vi "FrontPanel_RT.vi"() -> ()   [LabVIEW 2015]
uses:
  Classes/MotorControl/TypeDef/MotorMode.ctl
  Classes/CAlex2-Display/CAlex2_Display.lvclass
  Classes/CAlex2/TypeDef/LowerBodyDim.ctl
  Classes/ForceField/TypeDef/FF_Gains.ctl
  Classes/MotorControl/MotorControl.lvclass
  Classes/CAlex2/CAlex2.lvclass
  Classes/SerialChain-Cable/SerialChain-Cable.lvclass
  Classes/ForceField/ForceField.lvclass
  <vilib>/GoldZinc Software/auzn custom VIs/CustomVI.lvlib
panel:
  in  "Motor Mode":T1={"Idle"=FALSE, "Pre"=FALSE, "Pre-Value"=7, "PID"=FALSE} {"Pre-Value" items=["7N"=7, "10N"=10, "15N"=15, "20N"=20]}
  out "ViconConnected":bool
  in  "ResetIMU":bool
  in  "Vicon":bool
  in  "Extra Wt (kg)":cluster{"Thigh":dbl, "Shank":dbl}
  in  "UpdateFF":bool
  in  "XZ":bool
  in  "YZ":bool
  in  "XY":bool
  out "R_Hill":u32(colorbox)
  out "R_Ball":u32(colorbox)
  out "R_Toe":u32(colorbox)
  out "L_Hill":u32(colorbox)
  out "L_Ball":u32(colorbox)
  out "L_Toe":u32(colorbox)
  in  "Status 8":bool
  out "Waveform Chart 8":cluster{"[0]":dbl, "[1]":dbl}(graph)
  in  "Cuff Location":T2={"HipWd"=0.4, "HipHt"=0.1, "ThighDist"=0.0, "ThighToKnee"=0.05, "HipFwd"=0.0, "ShankToKnee"=0.15}
  in  "Force Field":bool
  in  "ArmWeight":bool
  in  "CuffWeight":bool
  out "Normal Force Tunnel Shape":cluster{dbl[], dbl[]}[](graph)
  in  "File Name":string
  out "Record Time":dbl format="%.2f"
  in  "Leg Property":T3={"Thigh"=0.42, "Shank"=0.42, "ShankWt"=0.0, "ThighWt"=0.0, "Hip"=0.32}
  in  "Gains":T4
  in  "Reset":bool
  in  "Stop RT":bool
  in  "Status 7":bool
  in  "Status 6":bool
  in  "Status 5":bool
  in  "Status 4":bool
  in  "Status 3":bool
  in  "Status 2":bool
  in  "Status 1":bool
  out "Waveform Chart 7":cluster{"[0]":dbl, "[1]":dbl}(graph)
  out "Waveform Chart 6":cluster{"[0]":dbl, "[1]":dbl}(graph)
  out "Waveform Chart 5":cluster{"[0]":dbl, "[1]":dbl}(graph)
  out "Waveform Chart 4":cluster{"[0]":dbl, "[1]":dbl}(graph)
  out "Waveform Chart 3":cluster{"[0]":dbl, "[1]":dbl}(graph)
  out "Waveform Chart 2":cluster{"[0]":dbl, "[1]":dbl}(graph)
  out "Waveform Chart":cluster{"[0]":dbl, "[1]":dbl}(graph)
  in  "ZeroPosition":bool
  in  "Path Type":u8(ring) items=["Straight Line", "Circle", "Vertical Wall", "Horizontal Surface", "Endoscope"]
  in  "Record Data?":bool
  out "Planned Tensions":dbl[](array[numeric]) format="%.2f"
  out "Motor Command":dbl[](array[numeric]) format="%.5f"
  out "Ankle Center":dbl[](array[numeric]) format="%.4f"
  out "Force Field":dbl[](array[numeric]) format="%.2f"
  out "Joint Angles":dbl[](array[numeric]) format="%.1f"
  in  "TareIMU":bool
  in  "Leg Position":refnum<k7>(container)
  # "C-ALEX Control Interface V2 \nDeveloped by Xin Jin, ROAR Laboratory, Columbia University"
  # "Leg Pose"
  # "Status Monitor"
  # "Subject Information"
  # "Data Record"
  # "Control Panel"
  # "Foot Switch"
  # "Path Type"
  # "Motor Mode"
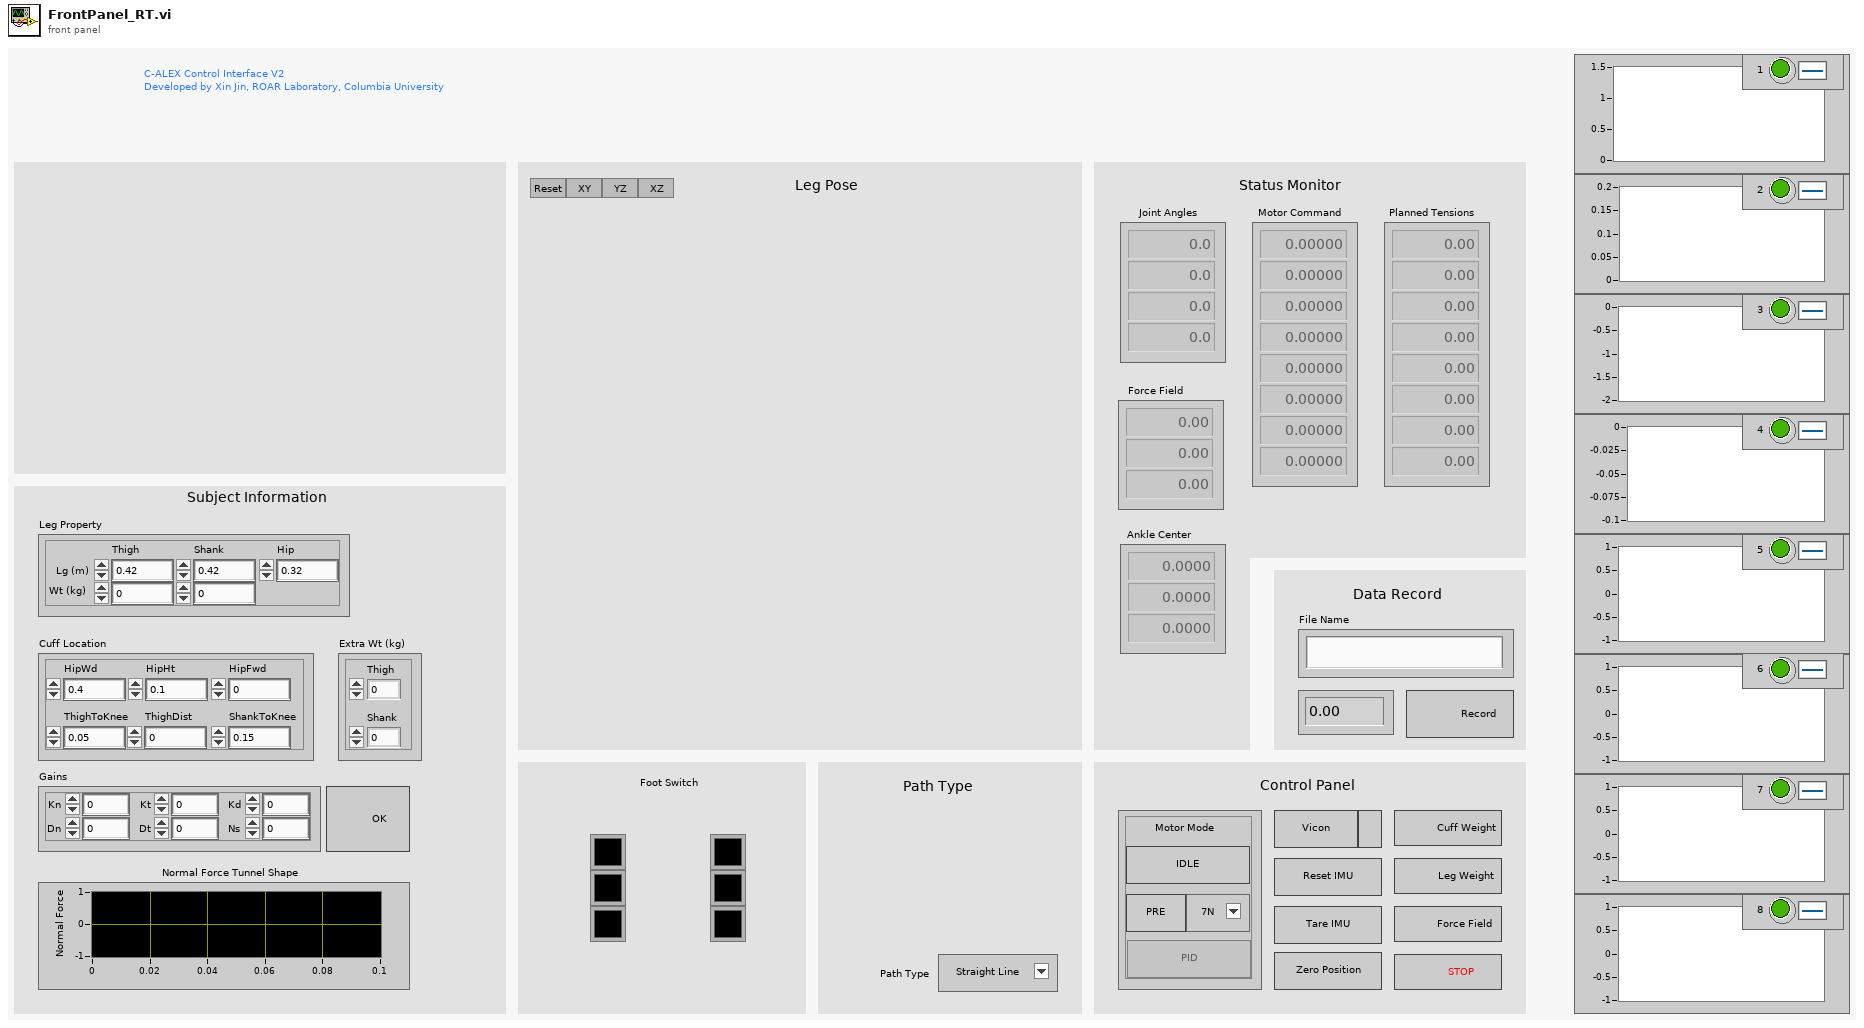
[diagram p1: front panel]
types:
  T1 = cluster{"Idle":bool, "Pre":bool, "Pre-Value":u8, "PID":bool}
  T2 = cluster{"HipWd":dbl, "HipHt":dbl, "ThighDist":dbl, "ThighToKnee":dbl, "HipFwd":dbl, "ShankToKnee":dbl}
  T3 = cluster{"Thigh":dbl, "Shank":dbl, "ShankWt":dbl, "ThighWt":dbl, "Hip":dbl}
  T4 = cluster{"Kn":dbl, "Dn":dbl, "Kt":dbl, "Dt":dbl, "Kd":dbl, "Ns":dbl}
  T5 = enum8{"Enabled", "Disabled", "Disabled and Grayed Out"}
  T6 = typedef "MotorControl.lvclass/MotorMode.ctl" = enum16{"Idle", "FF", "PID"}
  T7 = cluster{"AxisLabel":string[], "AxisMax":dbl[], "AxisMin":dbl[]}
  T8 = typedef "ForceField.lvclass/FF_Gains.ctl" = cluster{"Kn":dbl, "Dn":dbl, "Kt":dbl, "Dt":dbl, "Kd":dbl, "Ns":dbl}
  T9 = typedef "CAlex2.lvclass/LowerBodyDim.ctl" = cluster{"BodyDim(m)":cluster{"ThighLt":dbl, "ShankLt":dbl, "HipWd":dbl}, "BodyWt(kg)":cluster{"Thigh":dbl, "Shank":dbl}, "CuffLoc(m)":cluster{"HipCuffWd":dbl, "HipCuffHt":dbl, "HipCuffFwdShift":dbl, "ThighCuffToKnee":dbl, "ThighCuffDist":dbl, "ShankCuffToKnee":dbl}}
  T10 = cluster{"Input":enum16{"Fr:Cable", "Fr:Motor", "Fr:Sensor"}, "Output":enum16{"To:Cable", "To:Motor", "To:Sensor"}}
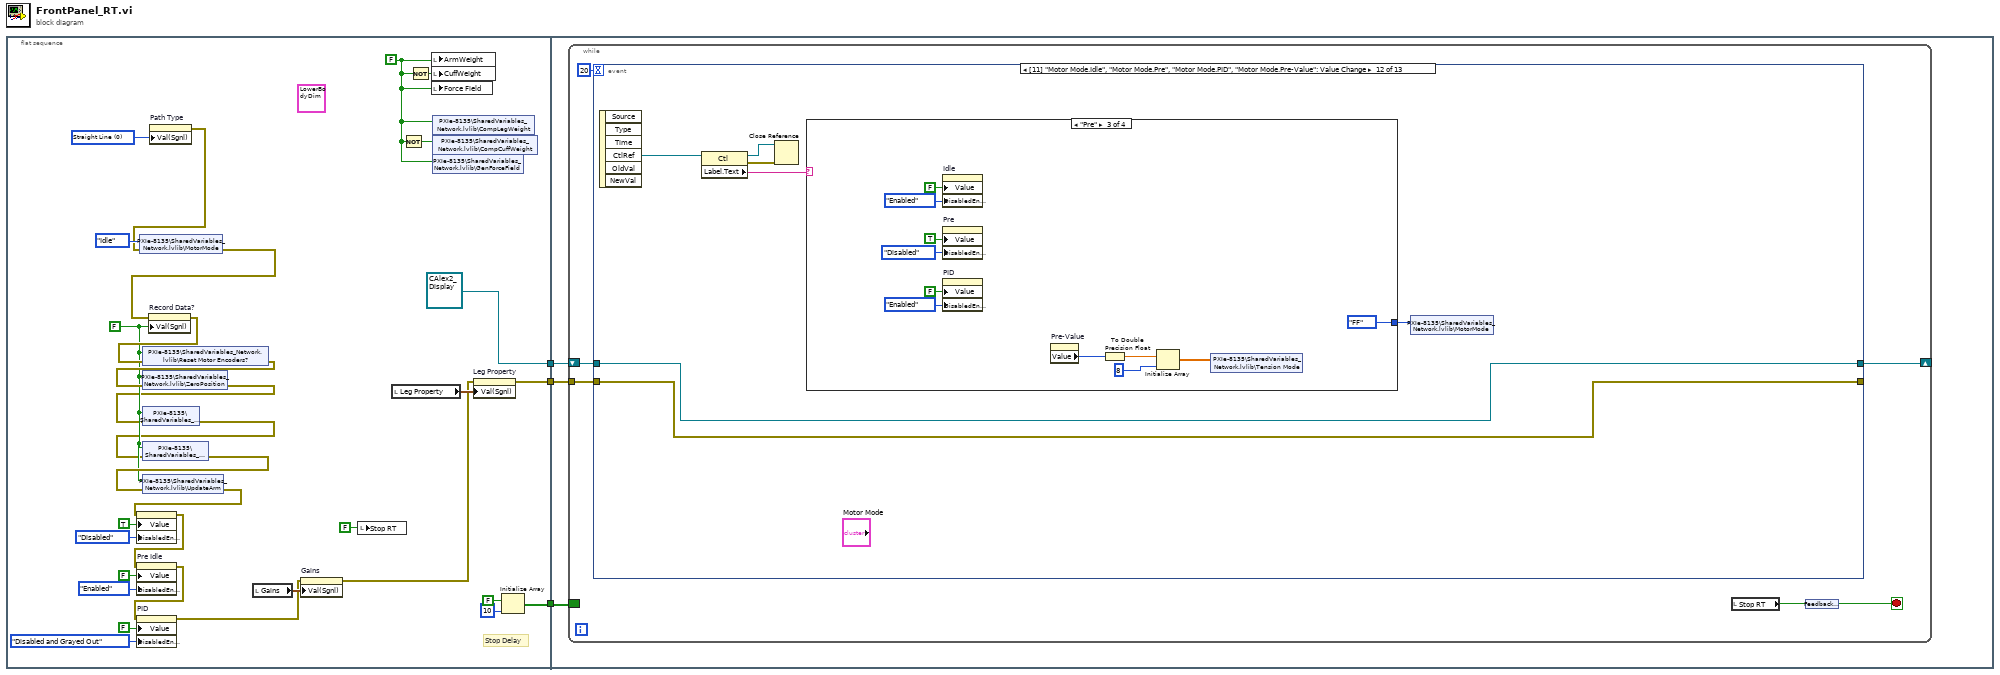
[diagram p0: block diagram]
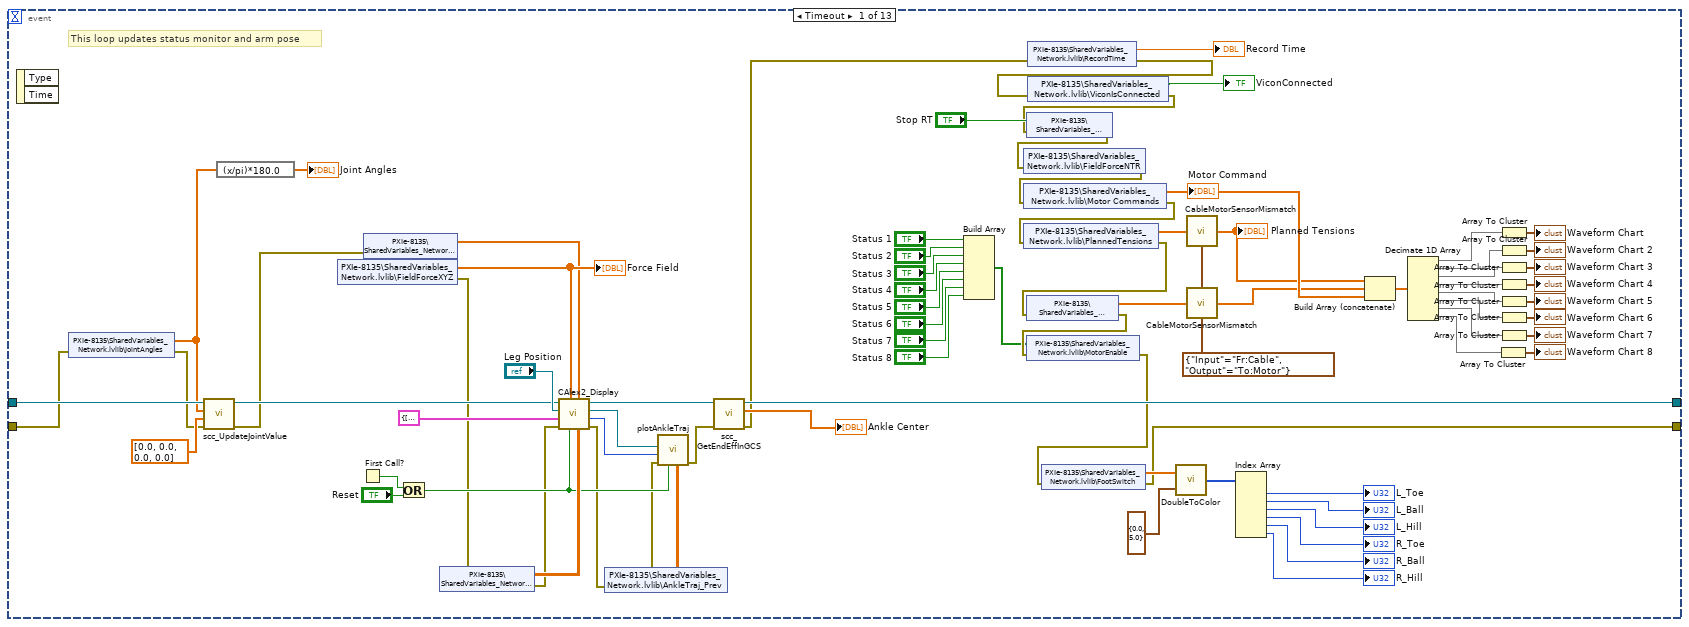
[diagram p2: hidden frame]
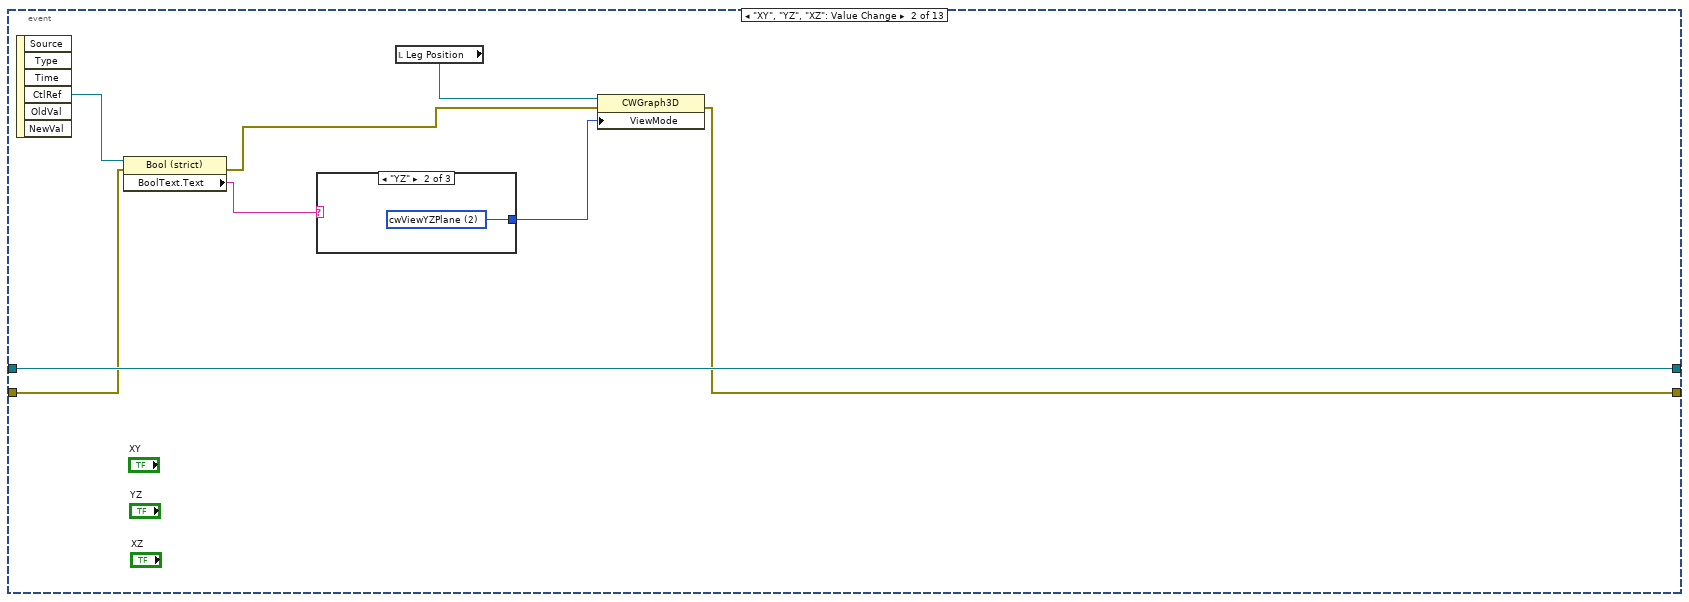
[diagram p3: hidden frame]
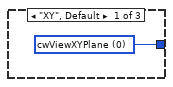
[diagram p4: hidden frame]
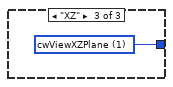
[diagram p5: hidden frame]
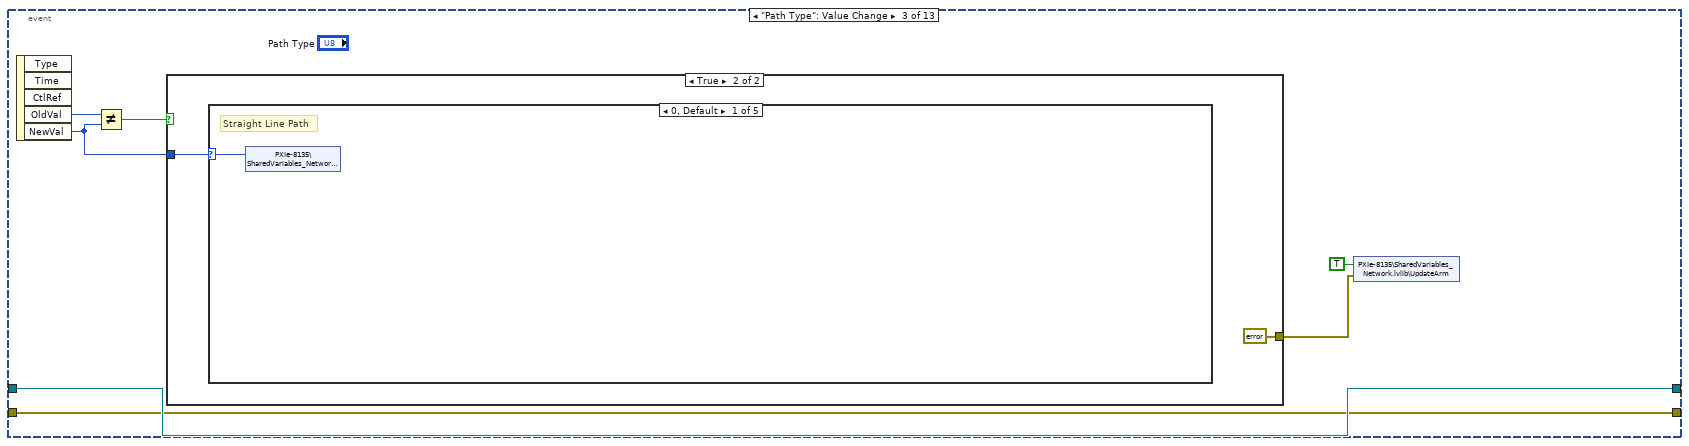
[diagram p6: hidden frame]
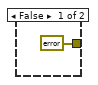
[diagram p7: hidden frame]
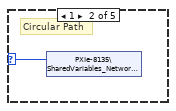
[diagram p8: hidden frame]
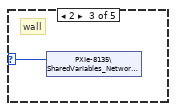
[diagram p9: hidden frame]
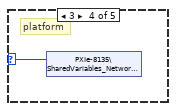
[diagram p10: hidden frame]
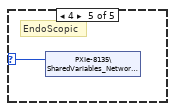
[diagram p11: hidden frame]
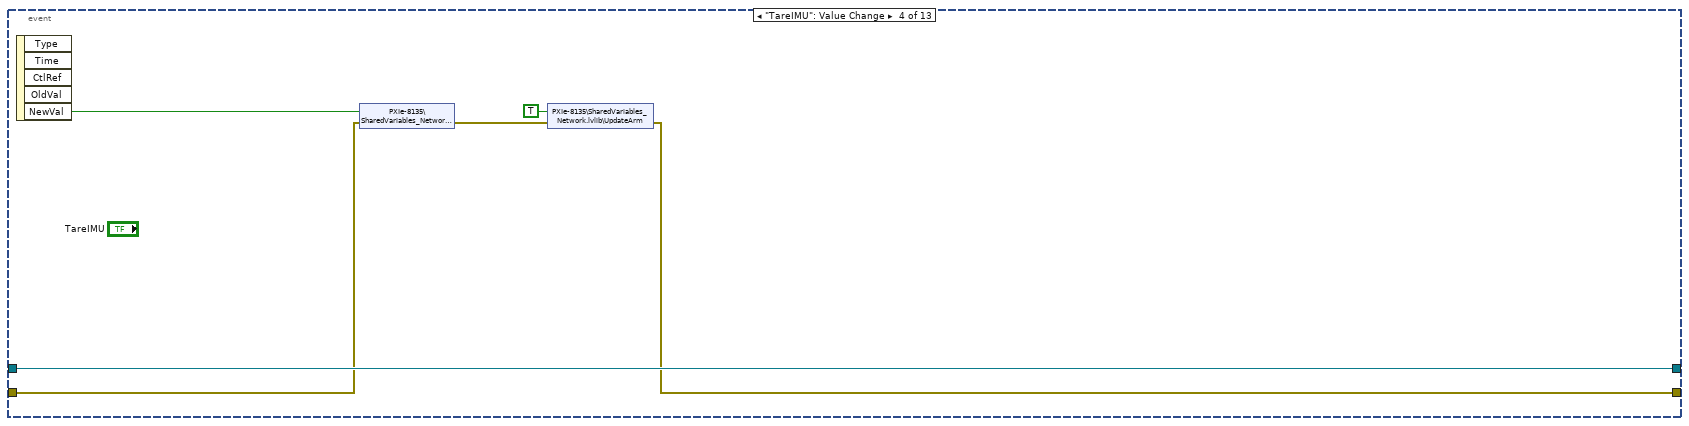
[diagram p12: hidden frame]
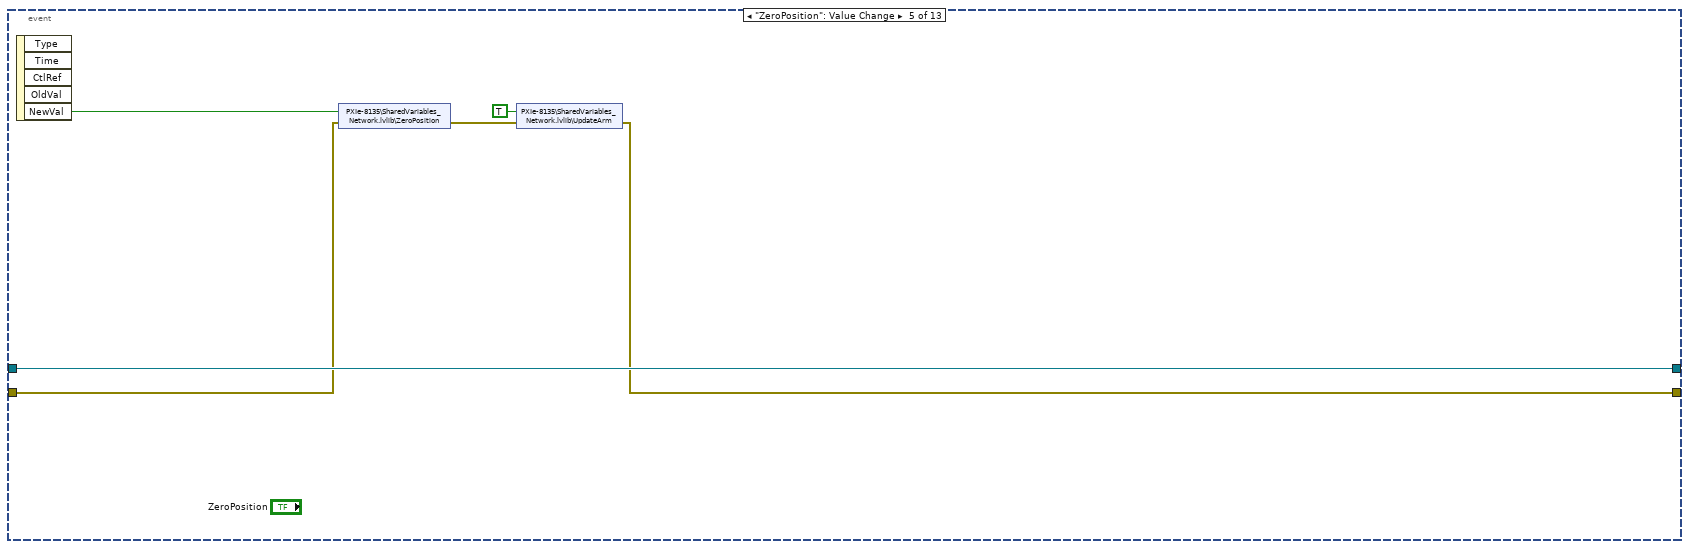
[diagram p13: hidden frame]
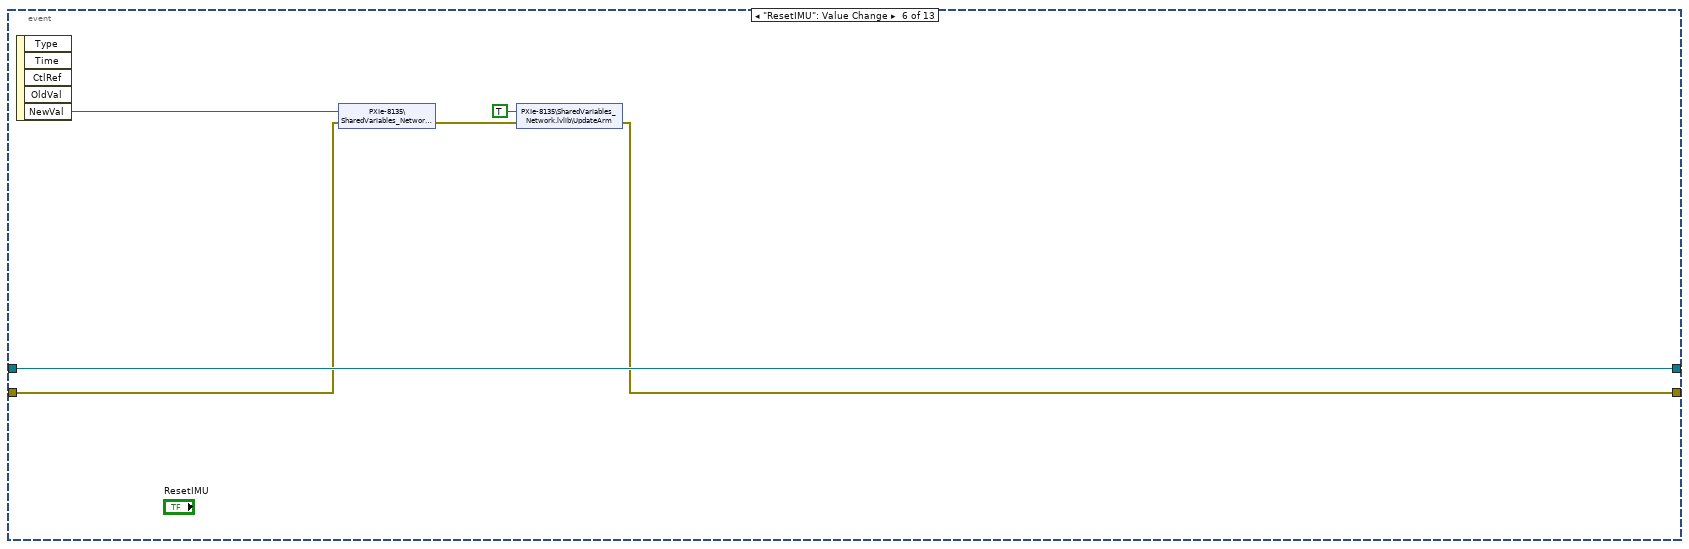
[diagram p14: hidden frame]
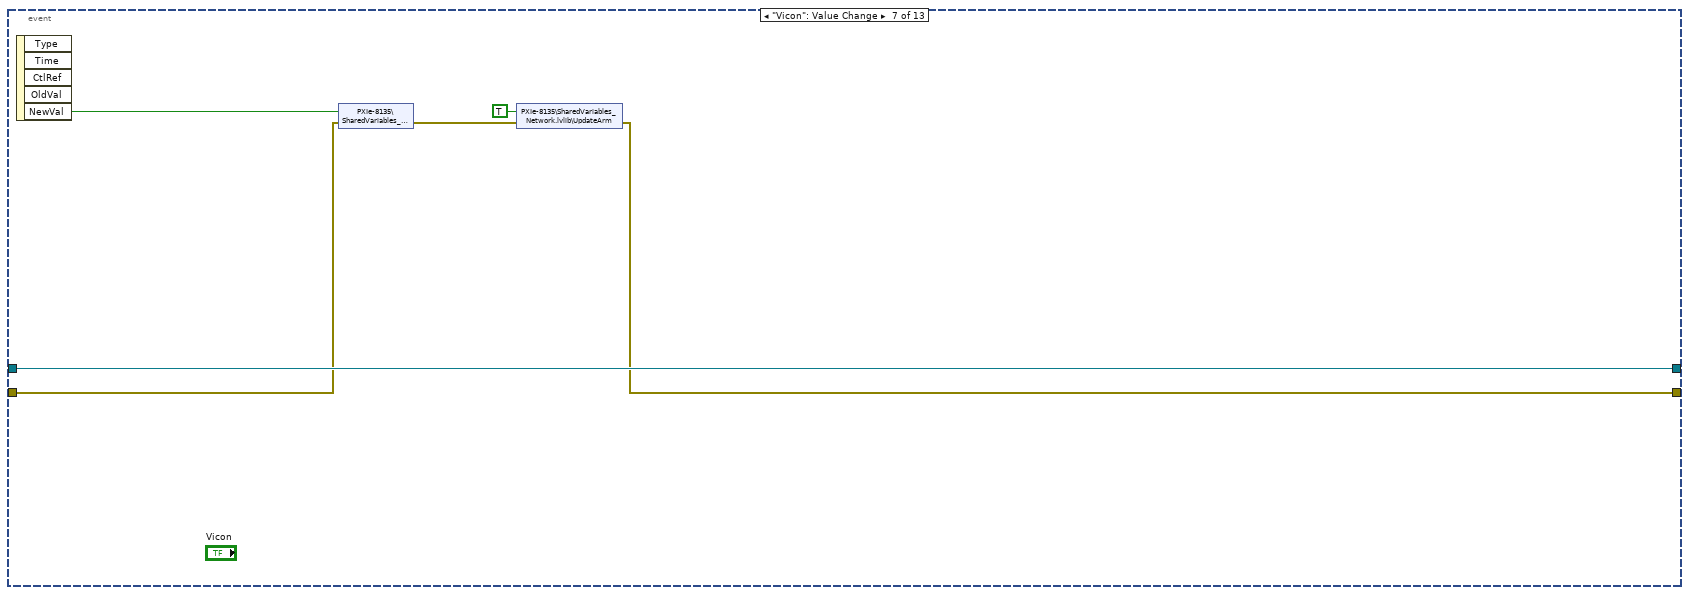
[diagram p15: hidden frame]
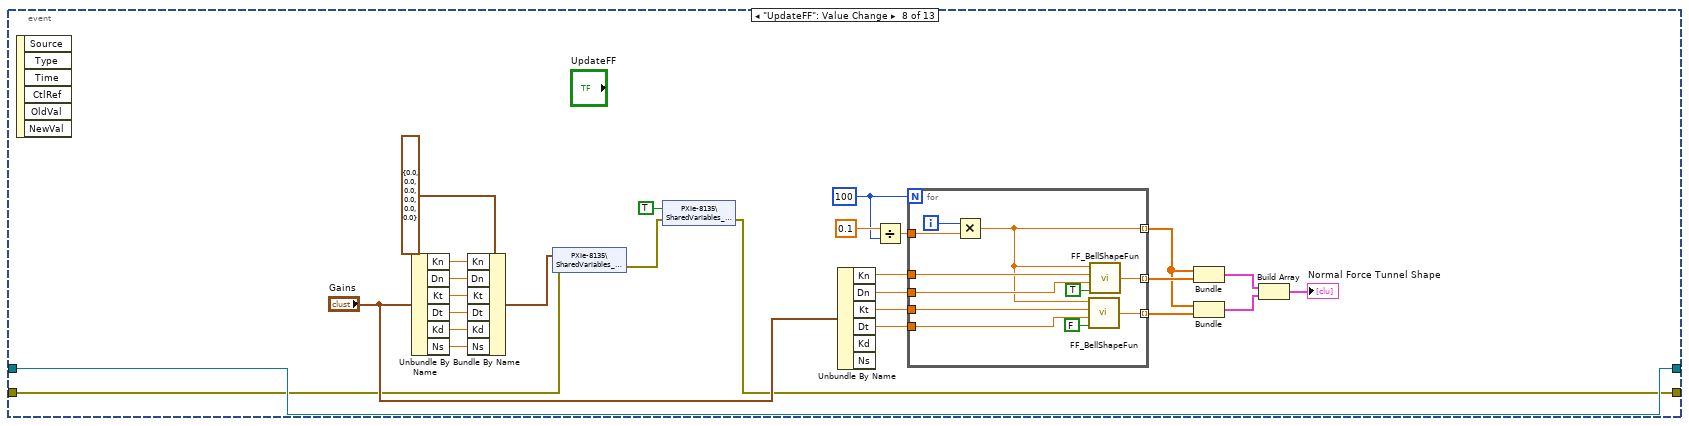
[diagram p16: hidden frame]
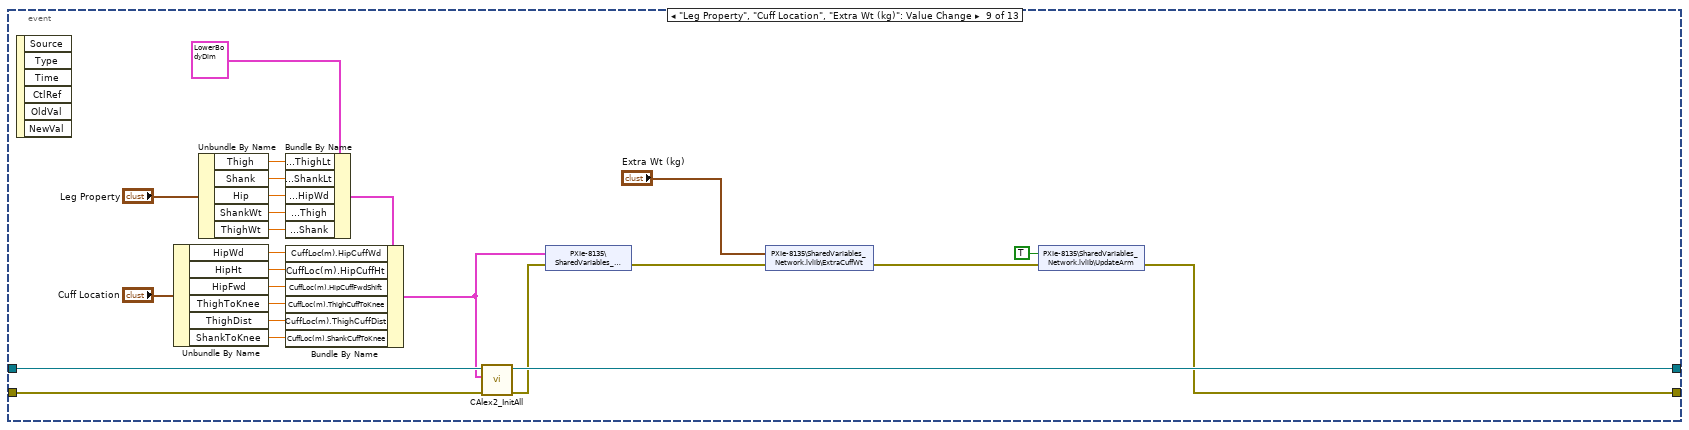
[diagram p17: hidden frame]
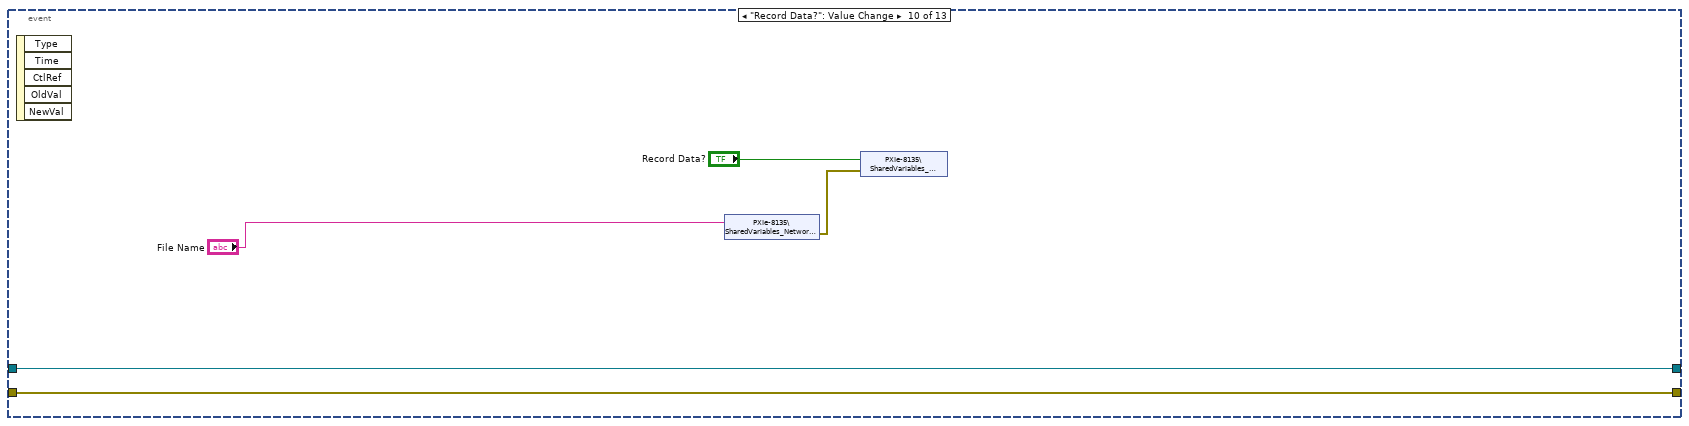
[diagram p18: hidden frame]
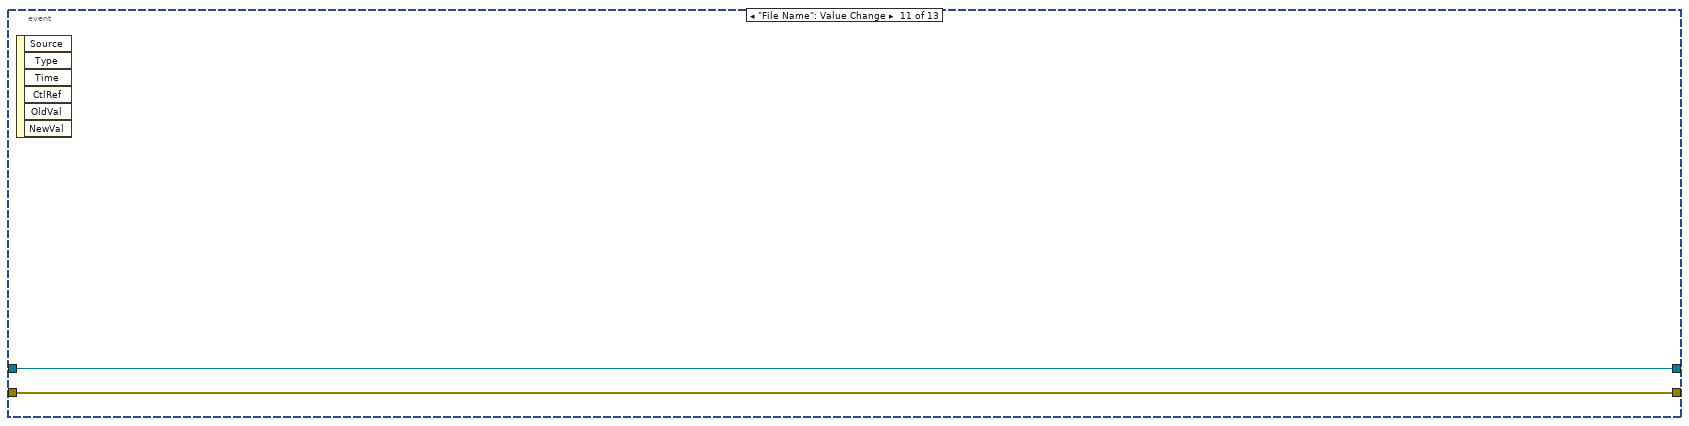
[diagram p19: hidden frame]
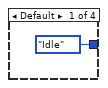
[diagram p20: hidden frame]
diagram:
  n1 = flat-sequence {
    tunnel: [w27] -> w3
    tunnel: [refnum<class "CAlex2_Display.lvclass"> refnum ("CAlex2")] -> w2
    tunnel: [w7] -> w1
    tunnel: w3 -> [w40]
    tunnel: w2 -> [w39]
    tunnel: w1 -> [w38]
    frame #0 {
      (unwired) T9 {"BodyDim(m)"={"ThighLt"=0.4, "ShankLt"=0.41, "HipWd"=0.32}, "BodyWt(kg)"={"Thigh"=0.0, "Shank"=0.0}, "CuffLoc(m)"={"HipCuffWd"=0.4, "HipCuffHt"=0.1, "HipCuffFwdShift"=0.0, "ThighCuffToKnee"=0.25, "ThighCuffDist"=0.0, "ShankCuffToKnee"=0.15}} ("LegProperties")
      w25 = u8 0 items=["Straight Line", "Circle", "Vertical Wall", "Horizontal Surface", "Endoscope"] ("Path Type")
      w32 = FALSE ("Es SH Center?")
      w6 = FALSE ("Es SH Center?")
      # "Stop Delay"
      n2 = property on="Path Type" class="Ring (strict)"("Val(Sgnl)"=w25) -> (error out=w24:errorcluster)  [unwired: 2 in, 1 out]
      n3 = shared-variable "PXIe-8135\\SharedVariables_Network.lvlib\\MotorMode"(MotorMode."Idle" ("MotorMode"), error in=w24) -> (error out=w23:errorcluster)
      n4 = property on="Record Data?" class="Bool (strict)"(error in=w23, "Val(Sgnl)"=w6) -> (error out=w22:errorcluster)  [unwired: 1 in, 1 out]
      n5 = shared-variable "PXIe-8135\\SharedVariables_Network.lvlib\\Reset Motor Encoders?"(w6, error in=w22) -> (error out=w36:errorcluster)
      n6 = shared-variable "PXIe-8135\\SharedVariables_Network.lvlib\\ZeroPosition"(w6, error in=w36) -> (error out=w5:errorcluster)
      n7 = shared-variable "PXIe-8135\\SharedVariables_Network.lvlib\\Vicon"(w6, error in=w5) -> (error out=w4:errorcluster)
      n8 = shared-variable "PXIe-8135\\SharedVariables_Network.lvlib\\Stop RT"(w6, error in=w4) -> (error out=w35:errorcluster)
      n9 = shared-variable "PXIe-8135\\SharedVariables_Network.lvlib\\UpdateArm"(w6, error in=w35) -> (error out=w13:errorcluster)
      n10 = property on="Idle" class="Bool (strict)"(error in=w13, "Value"=TRUE, "DisabledEnum"=T5."Disabled" ("Disabled")) -> (error out=w11:errorcluster)  [unwired: 1 in, 1 out]
      n11 = property on="Pre" class="Bool (strict)"(error in=w11, "Value"=FALSE, "DisabledEnum"=T5."Enabled" ("Disabled")) -> (error out=w10:errorcluster)  [unwired: 1 in, 1 out]
      n12 = property on="PID" class="Bool (strict)"(error in=w10, "Value"=FALSE, "DisabledEnum"=T5."Disabled and Grayed Out" ("Disabled")) -> (error out=w12:errorcluster)  [unwired: 1 in, 1 out]
      n13 = local read "Gains"() -> (w21:T4)
      n14 = property on="Gains" class="Clust (strict)"(error in=w12, "Val(Sgnl)"=w21) -> (error out=w20:errorcluster)  [unwired: 1 in, 1 out]
      n15 = local write "Stop RT"(FALSE ("Stop RT")) -> ()
      n16 = local read "Leg Property"() -> (w28:T3)
      n17 = Not(x=w32) -> (.not. x?=w33:bool)
      n18 = Not(x=w32) -> (.not. x?=w34:bool)
      n19 = local write "ArmWeight"(w32) -> ()
      n20 = local write "CuffWeight"(w34) -> ()
      n21 = local write "Force Field"(w32) -> ()
      n22 = shared-variable "PXIe-8135\\SharedVariables_Network.lvlib\\CompLegWeight"(w32) -> (error out=w31:errorcluster)  [unwired: 1 in]
      n23 = shared-variable "PXIe-8135\\SharedVariables_Network.lvlib\\CompCuffWeight"(w33, error in=w31) -> (error out=w30:errorcluster)
      n24 = shared-variable "PXIe-8135\\SharedVariables_Network.lvlib\\GenForceField"(w32, error in=w30) -> ()  [unwired: 1 out]
      n25 = property on="Leg Property" class="Clust (strict)"(error in=w20, "Val(Sgnl)"=w28) -> (error out=w27:errorcluster)  [unwired: 1 in, 1 out]
      n26 = Initialize Array(FALSE, 10 ("dimension size")) -> (w7:bool[])
    }
    frame #1 {
      n27 = while {
        tunnel: w40 -> [w44]
        shift-right: [w43] -> _
        shift-left: w39 -> [w45]
        border: w38 -> [_]
        stop <- w41 stop-if-true
        n28 = event shown="[11] \"Motor Mode.Idle\", \"Motor Mode.Pre\", \"Motor Mode.PID\", \"Motor Mode.Pre-Value\": Value Change" {
          selector: _ -> [_ _ _ _ _ _ _ _ _ _ _ _ _]
          dyn-events: _ -> [_ _ _ _ _ _ _ _ _ _ _ _ _]
          timeout: 20 -> [_ _ _ _ _ _ _ _ _ _ _ _ _]
          tunnel: [w54 w133 w140 w157 w164 w170 w176 w179 w236 w242 w247 w253 w285] -> _
          tunnel: w45 -> [w101 w136 w143 w160 w166 w172 w178 w205 w241 w246 w248 w255 w291]
          tunnel: w44 -> [w96 w130 w140 w158 w165 w171 w177 w180 w239 w242 w247 w253 w285]
          tunnel: [w99 w136 w143 w160 w166 w172 w178 w205 w240 w246 w248 w255 w291] -> w43
          event Timeout {
            w57 = T10 {"Input"=enum."Fr:Cable", "Output"=enum."To:Motor"} ("Conversion")
            # "This loop updates status monitor and arm pose"
            n29 = event-data() -> ()  [unwired: 1 in, 2 out]
            n30 = shared-variable "PXIe-8135\\SharedVariables_Network.lvlib\\JointAngles"(error in=w96) -> (w97:dbl[], error out=w95:errorcluster)
            n31 = call-dynamic "scc_UpdateJointValue.vi"("error in (no error)"=w95, "JointSpeed (rad|m|s)"=dbl[] [0.0, 0.0, 0.0, 0.0] ("JointSpeed (rad)"), "JointValue (rad|m)"=w97, "C-Alex in"=w101) -> ("error out"=w53:errorcluster, "C-Alex out"=w86:refnum<class "CAlex2_Display.lvclass">)  [unwired: 6 in]
            n32 = expression code="(x/pi)*180.0" ("radians to degrees")(w97) -> (→"Joint Angles":dbl[])
            n33 = First Call?() -> (First Call?: T/F=w102:bool)
            n34 = shared-variable "PXIe-8135\\SharedVariables_Network.lvlib\\ClosestPt"(error in=w53) -> (w79:dbl[], error out=w52:errorcluster)
            n35 = shared-variable "PXIe-8135\\SharedVariables_Network.lvlib\\FieldForceXYZ"(error in=w52) -> (w85:dbl[], error out=w51:errorcluster)
            "Force Field" <- w85
            n36 = Or(x=w102, y="Reset") -> (x .or. y?=w76:bool)
            n37 = shared-variable "PXIe-8135\\SharedVariables_Network.lvlib\\AnkleTraj"(error in=w51) -> (w80:dbl[][], error out=w50:errorcluster)
            n38 = call "CAlex2_Display.vi"("AnkleTraj"=w80, "ClosePt"=w79, "Init?"=w76, "Field Force"=w85, "error in (no error)"=w50, "AxisSetting"=T7 {"AxisLabel"=["x ", "y", "z "], "AxisMax"=[0.75, 0.3, 0.8], "AxisMin"=[-0.75, -1.2, -0.7]}, "3D graph in"="Leg Position", "CLX2 in"=w86) -> ("error out"=w49:errorcluster, "LastPlotNum"=w77:i32, "3D graph out"=w78:refnum<k7>, "CLX2 out"=w88:refnum<class "CAlex2_Display.lvclass">)
            n39 = shared-variable "PXIe-8135\\SharedVariables_Network.lvlib\\AnkleTraj_Prev"(error in=w49) -> (w75:dbl[][], error out=w56:errorcluster)
            n40 = call "plotAnkleTraj.vi"("AnkleTraj"=w75, "Init?"=w76, "error in (no error)"=w56, "PreviousPlotNum"=w77, "3D graph in"=w78) -> ("error out"=w47:errorcluster)  [unwired: 4 in, 2 out]
            n41 = call "scc_GetEndEffInGCS.vi"("error in (no error)"=w47, "SerialChain_Cable in"=w88) -> ("error out"=w48:errorcluster, "Pendeff(GCS)"=→"Ankle Center":dbl[], "SerialChain_Cable out"=w99:refnum<class "CAlex2_Display.lvclass">)  [unwired: 5 in, 2 out]
            n42 = Build Array("Status 1", "Status 2", "Status 3", "Status 4", "Status 5", "Status 6", "Status 7", "Status 8") -> (w104:bool[])
            n43 = shared-variable "PXIe-8135\\SharedVariables_Network.lvlib\\RecordTime"(error in=w48) -> (→"Record Time":dbl, error out=w62:errorcluster)
            n44 = shared-variable "PXIe-8135\\SharedVariables_Network.lvlib\\ViconIsConnected"(error in=w62) -> (→"ViconConnected":bool, error out=w65:errorcluster)
            n45 = shared-variable "PXIe-8135\\SharedVariables_Network.lvlib\\Stop RT"("Stop RT", error in=w65) -> (error out=w94:errorcluster)
            n46 = shared-variable "PXIe-8135\\SharedVariables_Network.lvlib\\FieldForceNTR"(error in=w94) -> (error out=w93:errorcluster)  [unwired: 1 out]
            n47 = shared-variable "PXIe-8135\\SharedVariables_Network.lvlib\\Motor Commands"(error in=w93) -> (w90:dbl[], error out=w128:errorcluster)
            "Motor Command" <- w90
            n48 = shared-variable "PXIe-8135\\SharedVariables_Network.lvlib\\PlannedTensions"(error in=w128) -> (w59:dbl[], error out=w92:errorcluster)
            n49 = shared-variable "PXIe-8135\\SharedVariables_Network.lvlib\\Tensions"(error in=w92) -> (w61:dbl[], error out=w112:errorcluster)
            n50 = shared-variable "PXIe-8135\\SharedVariables_Network.lvlib\\MotorEnable"(w104, error in=w112) -> (error out=w55:errorcluster)
            n51 = shared-variable "PXIe-8135\\SharedVariables_Network.lvlib\\FootSwitch"(error in=w55) -> (w74:dbl[], error out=w54:errorcluster)
            n52 = call <vilib>:"DoubleToColor.vi"("Value Range"=cluster{"ValueMin":dbl, "ValueMax":dbl} {"ValueMin"=0.0, "ValueMax"=5.0}, "Data"=w74) -> ("Colors"=w72:u32[])  [unwired: 1 in]
            n53 = call "CableMotorSensorMismatch.vi"("Conversion"=w57, "Input"=w59) -> ("Output"=w58:dbl[])  [unwired: 2 in]
            "Planned Tensions" <- w58
            n54 = call "CableMotorSensorMismatch.vi"("Conversion"=w57, "Input"=w61) -> ("Output"=w60:dbl[])  [unwired: 2 in]
            n55 = Index Array(array=w72) -> (element #1=→"L_Toe":u32, element #2=→"L_Ball":u32, element #3=→"L_Hill":u32, element #4=→"R_Toe":u32, element #5=→"R_Ball":u32, element #6=→"R_Hill":u32)  [unwired: 6 in]
            n56 = Build Array (concatenate)(w58, w60, w90) -> (w89:dbl[])
            n57 = Decimate 1D Array(w89) -> (w121:dbl[], w120:dbl[], w126:dbl[], w125:dbl[], w124:dbl[], w123:dbl[], w122:dbl[], w83:dbl[])
            n58 = Array To Cluster(array=w83) -> (cluster=→"Waveform Chart 8":cluster{"[0]":dbl, "[1]":dbl})
            n59 = Array To Cluster(array=w121) -> (cluster=→"Waveform Chart":cluster{"[0]":dbl, "[1]":dbl})
            n60 = Array To Cluster(array=w120) -> (cluster=→"Waveform Chart 2":cluster{"[0]":dbl, "[1]":dbl})
            n61 = Array To Cluster(array=w126) -> (cluster=→"Waveform Chart 3":cluster{"[0]":dbl, "[1]":dbl})
            n62 = Array To Cluster(array=w125) -> (cluster=→"Waveform Chart 4":cluster{"[0]":dbl, "[1]":dbl})
            n63 = Array To Cluster(array=w124) -> (cluster=→"Waveform Chart 5":cluster{"[0]":dbl, "[1]":dbl})
            n64 = Array To Cluster(array=w123) -> (cluster=→"Waveform Chart 6":cluster{"[0]":dbl, "[1]":dbl})
            n65 = Array To Cluster(array=w122) -> (cluster=→"Waveform Chart 7":cluster{"[0]":dbl, "[1]":dbl})
          }
          event "XY", "YZ", "XZ": Value Change {
            n66 = event-data() -> ("CtlRef"=w132:refnum<vi>)  [unwired: 1 in, 5 out]
            n67 = property class="Bool (strict)"(reference=w132, error in=w130) -> (error out=w131:errorcluster, "BoolText.Text"=w129:string)  [unwired: 1 out]
            n68 = case shown="\"YZ\"" w129 {
              tunnel: [w137 w138 w139] -> w134
              frame "XY", Default {
                w137 = 0 items=["cwViewXYPlane", "cwViewXZPlane", "cwViewYZPlane", "cwViewUserDefined"] ("ViewMode")
              }
              frame "YZ" {
                w138 = 2 items=["cwViewXYPlane", "cwViewXZPlane", "cwViewYZPlane", "cwViewUserDefined"] ("ViewMode")
              }
              frame "XZ" {
                w139 = 1 items=["cwViewXYPlane", "cwViewXZPlane", "cwViewYZPlane", "cwViewUserDefined"] ("ViewMode")
              }
            }
            n69 = local read "Leg Position"() -> (w135:refnum<k7>)
            n70 = property class="CWGraph3D"(reference=w135, error in=w131, "ViewMode"=w134) -> (error out=w133:errorcluster)  [unwired: 1 out]
          }
          event "Path Type": Value Change {
            n71 = event-data() -> ("OldVal"=w146:u8, "NewVal"=w144:u8)  [unwired: 1 in, 3 out]
            n72 = Not Equal?(x=w146, y=w144) -> (x != y?=w145:bool)
            n73 = case shown="True" w145 {
              tunnel: w144 -> [_ w149]
              tunnel: [errorcluster {"status"=FALSE, "code"=0, "source"=""} ("error IO") errorcluster {"status"=FALSE, "code"=0, "source"=""} ("error IO")] -> w141
              frame False {
              }
              frame True {
                n74 = case shown="0, Default" w149 {
                  selector: w149 -> [w150 w151 w152 w153 w154]
                  frame 0, Default {
                    # "Straight Line Path"
                    n75 = shared-variable "PXIe-8135\\SharedVariables_Network.lvlib\\PathType"(w150) -> ()  [unwired: 1 in, 1 out]
                  }
                  frame 1 {
                    # "Circular Path"
                    n76 = shared-variable "PXIe-8135\\SharedVariables_Network.lvlib\\PathType"(w151) -> ()  [unwired: 1 in, 1 out]
                  }
                  frame 2 {
                    # "wall"
                    n77 = shared-variable "PXIe-8135\\SharedVariables_Network.lvlib\\PathType"(w152) -> ()  [unwired: 1 in, 1 out]
                  }
                  frame 3 {
                    # "platform"
                    n78 = shared-variable "PXIe-8135\\SharedVariables_Network.lvlib\\PathType"(w153) -> ()  [unwired: 1 in, 1 out]
                  }
                  frame 4 {
                    # "EndoScopic"
                    n79 = shared-variable "PXIe-8135\\SharedVariables_Network.lvlib\\PathType"(w154) -> ()  [unwired: 1 in, 1 out]
                  }
                }
              }
            }
            n80 = shared-variable "PXIe-8135\\SharedVariables_Network.lvlib\\UpdateArm"(TRUE ("UpdateArm"), error in=w141) -> ()  [unwired: 1 out]
          }
          event "TareIMU": Value Change {
            n81 = event-data() -> ("NewVal"=w159:bool)  [unwired: 1 in, 4 out]
            n82 = shared-variable "PXIe-8135\\SharedVariables_Network.lvlib\\IMU_Tare"(w159, error in=w158) -> (error out=w155:errorcluster)
            n83 = shared-variable "PXIe-8135\\SharedVariables_Network.lvlib\\UpdateArm"(TRUE ("UpdateArm"), error in=w155) -> (error out=w157:errorcluster)
          }
          event "ZeroPosition": Value Change {
            n84 = event-data() -> ("NewVal"=w163:bool)  [unwired: 1 in, 4 out]
            n85 = shared-variable "PXIe-8135\\SharedVariables_Network.lvlib\\ZeroPosition"(w163, error in=w165) -> (error out=w161:errorcluster)
            n86 = shared-variable "PXIe-8135\\SharedVariables_Network.lvlib\\UpdateArm"(TRUE ("UpdateArm"), error in=w161) -> (error out=w164:errorcluster)
          }
          event "ResetIMU": Value Change {
            n87 = event-data() -> ("NewVal"=w169:bool)  [unwired: 1 in, 4 out]
            n88 = shared-variable "PXIe-8135\\SharedVariables_Network.lvlib\\IMU_reset"(w169, error in=w171) -> (error out=w167:errorcluster)
            n89 = shared-variable "PXIe-8135\\SharedVariables_Network.lvlib\\UpdateArm"(TRUE ("UpdateArm"), error in=w167) -> (error out=w170:errorcluster)
          }
          event "Vicon": Value Change {
            n90 = event-data() -> ("NewVal"=w175:bool)  [unwired: 1 in, 4 out]
            n91 = shared-variable "PXIe-8135\\SharedVariables_Network.lvlib\\Vicon"(w175, error in=w177) -> (error out=w173:errorcluster)
            n92 = shared-variable "PXIe-8135\\SharedVariables_Network.lvlib\\UpdateArm"(TRUE ("UpdateArm"), error in=w173) -> (error out=w176:errorcluster)
          }
          event "UpdateFF": Value Change {
            w190 = 100
            n93 = event-data() -> ()  [unwired: 1 in, 6 out]
            n94 = Unbundle By Name("Gains") -> ("Kn"=w204:dbl, "Dn"=w202:dbl, "Kt"=w201:dbl, "Dt"=w200:dbl, "Kd"=w199:dbl, "Ns"=w198:dbl)
            n95 = Bundle By Name(cluster=T8 {"Kn"=0.0, "Dn"=0.0, "Kt"=0.0, "Dt"=0.0, "Kd"=0.0, "Ns"=0.0} ("Gains"), "Kn"=w204, "Dn"=w202, "Kt"=w201, "Dt"=w200, "Kd"=w199, "Ns"=w198) -> (w197:T8)
            n96 = shared-variable "PXIe-8135\\SharedVariables_Network.lvlib\\Gains"(w197, error in=w180) -> (error out=w181:errorcluster)
            n97 = shared-variable "PXIe-8135\\SharedVariables_Network.lvlib\\FFRst"(TRUE ("UpdateArm"), error in=w181) -> (error out=w179:errorcluster)
            n98 = Unbundle By Name("Gains") -> ("Kn"=w195:dbl, "Dn"=w194:dbl, "Kt"=w193:dbl, "Dt"=w192:dbl)  [unwired: 2 out]
            n99 = Divide(x=0.1, y=w190) -> (x/y=w189:dbl)
            n100 = for {
              N: w190 -> [_]
              tunnel: w195 -> [w216]
              tunnel: w194 -> [w215]
              tunnel: w193 -> [w214]
              tunnel: w192 -> [w213]
              tunnel: w189 -> [w209]
              tunnel: [w208] -> w186 mode=indexing
              tunnel: [w207] -> w187 mode=indexing
              tunnel: [w206] -> w188 mode=indexing
              i -> [w210]
              n101 = Multiply(x=w210, y=w209) -> (x*y=w208:dbl)
              n102 = call "FF_BellShapeFun.vi"("Invert(F)"=FALSE, "(r)adius"=w213, "(A)mplitude"=w214, "x"=w208) -> ("y"=w206:dbl)  [unwired: 2 in]
              n103 = call "FF_BellShapeFun.vi"("Invert(F)"=TRUE ("Invert"), "(r)adius"=w215, "(A)mplitude"=w216, "x"=w208) -> ("y"=w207:dbl)  [unwired: 2 in]
            }
            n104 = Bundle(w186, w187) -> (w184:cluster{dbl[], dbl[]})  [unwired: 1 in]
            n105 = Bundle(w186, w188) -> (w185:cluster{dbl[], dbl[]})  [unwired: 1 in]
            n106 = Build Array(w184, w185) -> (→"Normal Force Tunnel Shape":cluster{dbl[], dbl[]}[])
          }
          event "Leg Property", "Cuff Location", "Extra Wt (kg)": Value Change {
            n107 = event-data() -> ()  [unwired: 1 in, 6 out]
            n108 = Unbundle By Name("Cuff Location") -> ("HipWd"=w225:dbl, "HipHt"=w224:dbl, "HipFwd"=w223:dbl, "ThighToKnee"=w222:dbl, "ThighDist"=w221:dbl, "ShankToKnee"=w220:dbl)
            n109 = Unbundle By Name("Leg Property") -> ("Thigh"=w231:dbl, "Shank"=w232:dbl, "Hip"=w233:dbl, "ShankWt"=w234:dbl, "ThighWt"=w235:dbl)
            n110 = Bundle By Name(cluster=T9 {"BodyDim(m)"={"ThighLt"=0.4, "ShankLt"=0.41, "HipWd"=0.32}, "BodyWt(kg)"={"Thigh"=0.0, "Shank"=0.0}, "CuffLoc(m)"={"HipCuffWd"=0.4, "HipCuffHt"=0.1, "HipCuffFwdShift"=0.0, "ThighCuffToKnee"=0.25, "ThighCuffDist"=0.0, "ShankCuffToKnee"=0.15}} ("LegProperties"), "BodyDim(m).ThighLt"=w231, "BodyDim(m).ShankLt"=w232, "BodyDim(m).HipWd"=w233, "BodyWt(kg).Thigh"=w234, "BodyWt(kg).Shank"=w235) -> (w228:T9)
            n111 = Bundle By Name(cluster=w228, "CuffLoc(m).HipCuffWd"=w225, "CuffLoc(m).HipCuffHt"=w224, "CuffLoc(m).HipCuffFwdShift"=w223, "CuffLoc(m).ThighCuffToKnee"=w222, "CuffLoc(m).ThighCuffDist"=w221, "CuffLoc(m).ShankCuffToKnee"=w220) -> (w227:T9)
            n112 = call-dynamic "CAlex2_InitAll.vi"("error in (no error)"=w239, "LegProperties"=w227, "CAlex2 in"=w241) -> ("error out"=w238:errorcluster, "CAlex2 out"=w240:refnum<class "CAlex2_Display.lvclass">)  [unwired: 7 in]
            n113 = shared-variable "PXIe-8135\\SharedVariables_Network.lvlib\\LegDim"(w227, error in=w238) -> (error out=w218:errorcluster)
            n114 = shared-variable "PXIe-8135\\SharedVariables_Network.lvlib\\ExtraCuffWt"("Extra Wt (kg)", error in=w218) -> (error out=w217:errorcluster)
            n115 = shared-variable "PXIe-8135\\SharedVariables_Network.lvlib\\UpdateArm"(TRUE ("UpdateArm"), error in=w217) -> (error out=w236:errorcluster)
          }
          event "Record Data?": Value Change {
            n116 = event-data() -> ()  [unwired: 1 in, 5 out]
            n117 = shared-variable "PXIe-8135\\SharedVariables_Network.lvlib\\FileName"("File Name") -> (error out=w244:errorcluster)  [unwired: 1 in]
            n118 = shared-variable "PXIe-8135\\SharedVariables_Network.lvlib\\Record?"("Record Data?", error in=w244) -> ()  [unwired: 1 out]
          }
          event "File Name": Value Change {
            n119 = event-data() -> ()  [unwired: 1 in, 6 out]
          }
          event "Motor Mode.Idle", "Motor Mode.Pre", "Motor Mode.PID", "Motor Mode.Pre-Value": Value Change {
            n120 = event-data() -> ("CtlRef"=w252:refnum<vi>)  [unwired: 1 in, 5 out]
            n121 = property class="Ctl"(reference=w252) -> (reference out=w249:refnum<vi>, error out=w250:errorcluster, "Label.Text"=w251:string)  [unwired: 1 in]
            n122 = Close Reference(reference=w249, error in (no error)=w250) -> ()  [unwired: 1 out]
            n123 = case shown="\"Pre\"" w251 {
              tunnel: [MotorMode."Idle" ("MotorMode") MotorMode."Idle" ("MotorMode") MotorMode."FF" ("MotorMode") MotorMode."PID" ("MotorMode")] -> w254
              frame Default {
              }
              frame "Idle" {
                n124 = property on="Idle" class="Bool (strict)"("Value"=TRUE, "DisabledEnum"=T5."Disabled" ("Disabled")) -> ()  [unwired: 2 in, 2 out]
                n125 = property on="Pre" class="Bool (strict)"("Value"=FALSE, "DisabledEnum"=T5."Enabled" ("Disabled")) -> ()  [unwired: 2 in, 2 out]
                n126 = property on="PID" class="Bool (strict)"("Value"=FALSE, "DisabledEnum"=T5."Disabled and Grayed Out" ("Disabled")) -> ()  [unwired: 2 in, 2 out]
                n127 = Initialize Array(0.0 ("element"), 8 ("dimension size")) -> (w264:dbl[])
                n128 = shared-variable "PXIe-8135\\SharedVariables_Network.lvlib\\Tension Mode"(w264) -> ()  [unwired: 1 in, 1 out]
              }
              frame "Pre" {
                n129 = property on="Idle" class="Bool (strict)"("Value"=FALSE, "DisabledEnum"=T5."Enabled" ("Disabled")) -> ()  [unwired: 2 in, 2 out]
                n130 = property on="Pre" class="Bool (strict)"("Value"=TRUE, "DisabledEnum"=T5."Disabled" ("Disabled")) -> ()  [unwired: 2 in, 2 out]
                n131 = property on="PID" class="Bool (strict)"("Value"=FALSE, "DisabledEnum"=T5."Enabled" ("Disabled")) -> ()  [unwired: 2 in, 2 out]
                n132 = property on="Pre-Value" class="Ring (strict)"() -> ("Value"=w271:u8)  [unwired: 2 in, 2 out]
                n133 = To Double Precision Float(number=w271) -> (double precision float=w270:dbl)
                n134 = Initialize Array(w270, 8 ("dimension size")) -> (w275:dbl[])
                n135 = shared-variable "PXIe-8135\\SharedVariables_Network.lvlib\\Tension Mode"(w275) -> ()  [unwired: 1 in, 1 out]
              }
              frame "PID" {
                n136 = property on="Idle" class="Bool (strict)"("Value"=FALSE, "DisabledEnum"=T5."Enabled" ("Disabled")) -> ()  [unwired: 2 in, 2 out]
                n137 = property on="Pre" class="Bool (strict)"("Value"=FALSE, "DisabledEnum"=T5."Disabled and Grayed Out" ("Disabled")) -> ()  [unwired: 2 in, 2 out]
                n138 = property on="PID" class="Bool (strict)"("Value"=TRUE, "DisabledEnum"=T5."Disabled" ("Disabled")) -> ()  [unwired: 2 in, 2 out]
              }
            }
            n139 = shared-variable "PXIe-8135\\SharedVariables_Network.lvlib\\MotorMode"(w254) -> ()  [unwired: 1 in, 1 out]
          }
          event "CuffWeight", "ArmWeight", "Force Field": Value Change {
            n140 = event-data() -> ()  [unwired: 1 in, 6 out]
            n141 = shared-variable "PXIe-8135\\SharedVariables_Network.lvlib\\CompLegWeight"("ArmWeight") -> (error out=w287:errorcluster)  [unwired: 1 in]
            n142 = shared-variable "PXIe-8135\\SharedVariables_Network.lvlib\\CompCuffWeight"("CuffWeight", error in=w287) -> (error out=w286:errorcluster)
            n143 = shared-variable "PXIe-8135\\SharedVariables_Network.lvlib\\GenForceField"("Force Field", error in=w286) -> ()  [unwired: 1 out]
          }
        }
        n144 = local read "Stop RT"() -> (w42:bool)
        n145 = feedback-in #1(w42) -> ()
        n146 = feedback #1() -> (w41:bool)
      }
    }
  }
